vi "Acquire Data.vi"(6 "MemberAttendance":refnum<class "MemberAttendance.lvclass">, 8 "error in (no error)":errorcluster, 9 "ExcuseNote":refnum<class "ExcuseNote.lvclass">, 10 "TimeTable":refnum<class "TimeTable.lvclass">, 11 "CalAttendance in":refnum<class "CalAttendance.lvclass">) -> (0 "error out":errorcluster, 3 "CalAttendance out":refnum<class "CalAttendance.lvclass">)   [LabVIEW 2015, in "Admin_Actor.lvlib" / "CalAttendance.lvclass"]
uses:
  CalAttendance.lvclass
  Member_Actor/MemberTable/TimeTable.lvclass
  Member_Actor/ExcuseNote/ExcuseNote.lvclass
  Models/MemberAttendance/MemberAttendance.lvclass
  CalAttendance.lvclass/CalAttendance.ctl
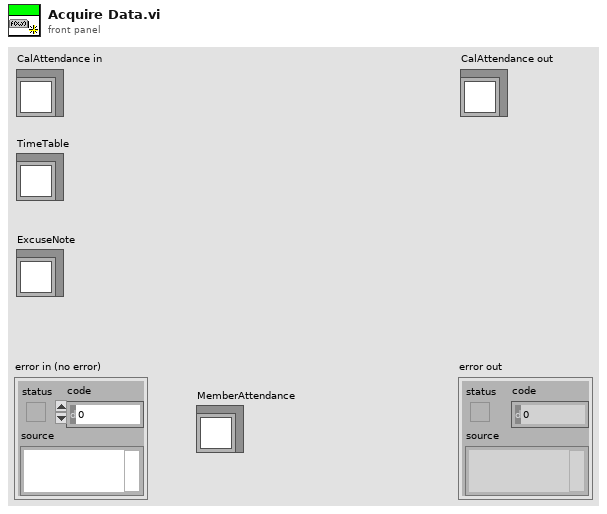
[diagram p1: front panel]
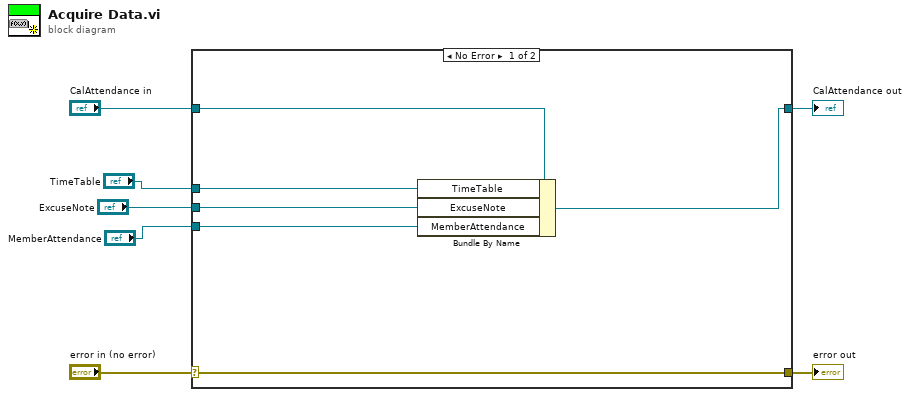
[diagram p0: block diagram]
diagram:
  n1 = case shown="No Error" "error in (no error)" {
    selector: "error in (no error)" -> [w13 w15]
    tunnel: [w13 w15] -> w6
    tunnel: [w11 w14] -> w4
    tunnel: "CalAttendance in" -> [w12 w14]
    tunnel: "TimeTable" -> [w10 _]
    tunnel: "ExcuseNote" -> [w9 _]
    tunnel: "MemberAttendance" -> [w8 _]
    frame No Error {
      n2 = Bundle By Name(cluster=w12, "TimeTable"=w10, "ExcuseNote"=w9, "MemberAttendance"=w8) -> (w11:refnum<class "CalAttendance.lvclass">)
    }
    frame Error {
    }
  }
  "error out" <- w6
  "CalAttendance out" <- w4
